vi "习3.4.vi"() -> ()   [LabVIEW 2017]
panel:
  out "长度":i32
  out "结果字符串":string
  in  "尾":string
  in  "头":string
  in  "数值 2":dbl
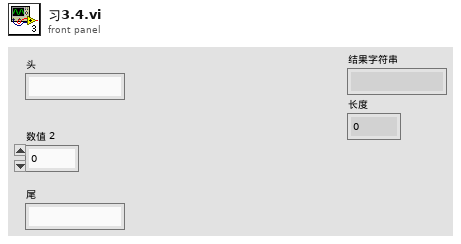
[diagram p1: front panel]
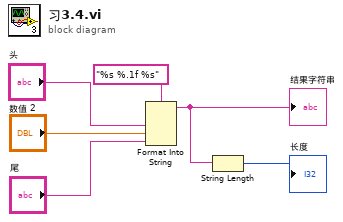
[diagram p0: block diagram]
diagram:
  n1 = Format Into String(format string="%s %.1f %s" ("格式字符串"), "头", "数值 2", "尾") -> (resulting string=w2:string)  [unwired: 2 in, 1 out]
  "结果字符串" <- w2
  n2 = String Length(string=w2) -> (length=→"长度":i32)
